vi "UI IDEX.vi"(8 "error in":errorcluster) -> (0 "error out":errorcluster)   [LabVIEW 2019, in "IDEX.lvlib"]
uses:
  IDEX.lvlib
  User Event/Controls/UE Abort Action.ctl
  <vilib>/Utility/miscctls.llb/LVPointTypeDef.ctl
  Queues/Queues.lvlib
panel:
  in  "Selection Valve":T1(ring)
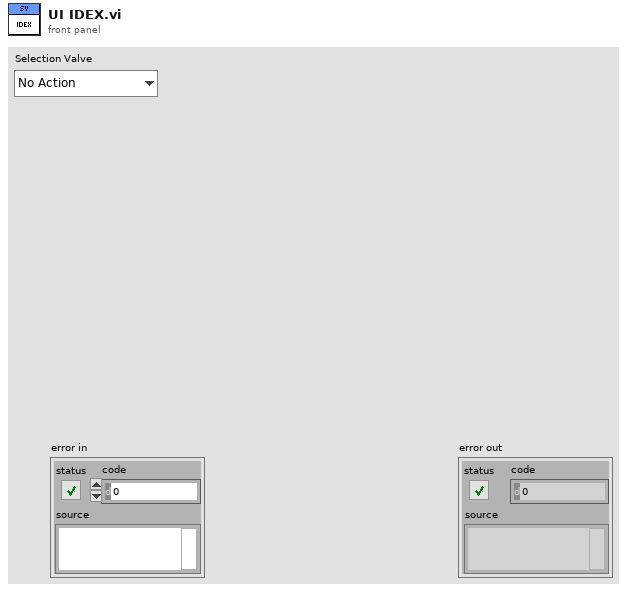
[diagram p1: front panel]
types:
  T1 = enum16{"No Action", "Position 1", "Position 2", "Position 3", "Position 4", "Position 5", "Position 6"}
  T2 = typedef "UE Abort Action.ctl" = enum16{"Create", "Get", "Destroy"}
  T3 = typedef "LVPointTypeDef.ctl" = cluster{"Horizontal":i16, "Vertical":i16}
  T4 = enum16{"Open", "Read", "Move", "Home", "Command", "Close"}
  T5 = typedef "IDEX.lvlib/SEQ Data.ctl" = cluster{"Position":string, "Initialize Done?":bool, "VI Refnum":refnum<vi>}
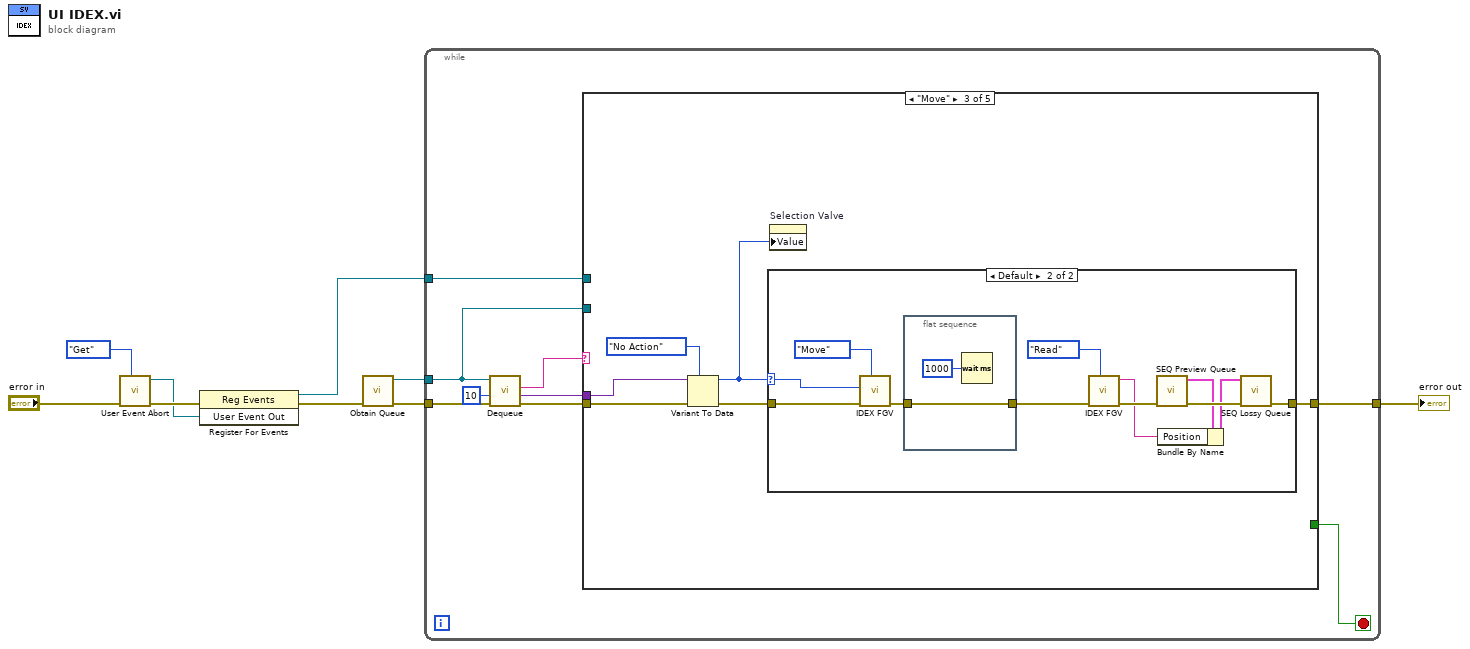
[diagram p0: block diagram]
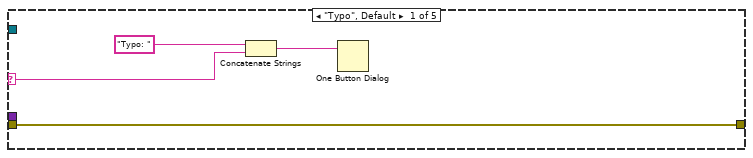
[diagram p2: hidden frame]
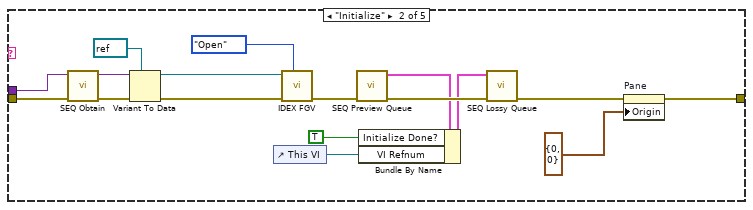
[diagram p3: hidden frame]
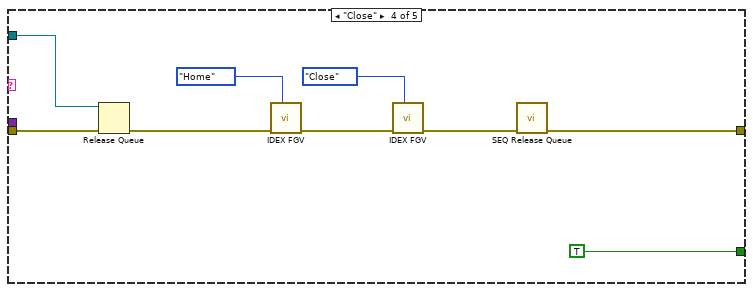
[diagram p5: hidden frame]
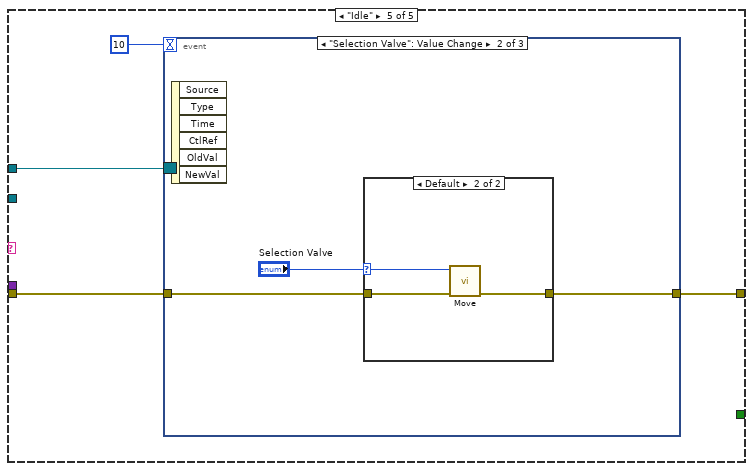
[diagram p6: hidden frame]
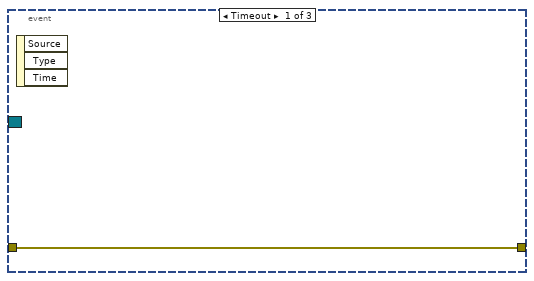
[diagram p7: hidden frame]
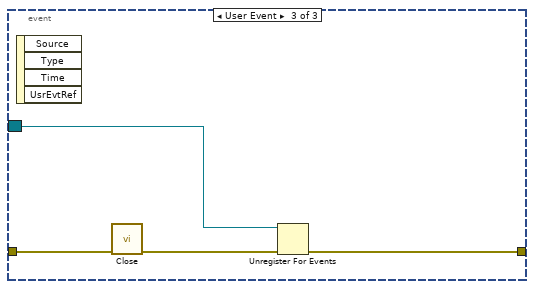
[diagram p9: hidden frame]
diagram:
  n1 = call "User Event Abort.vi"("Action"=UE_Abort_Action."Get", "Error In"="error in") -> ("Error Out"=w7:errorcluster, "User Event Out"=w6:refnum<user-event>)  [unwired: 8 in]
  n2 = register-events(error in=w7, w6) -> (reference out=w1:refnum<event-registration>, error out=w5:errorcluster)  [unwired: 1 in]
  n3 = call "Obtain Queue.vi"("Error In"=w5) -> ("Error Out"=w4:errorcluster, "Queue out"=w3:refnum<queue>)  [unwired: 9 in]
  n4 = while {
    tunnel: w4 -> [w18]
    tunnel: w3 -> [w13]
    tunnel: [w12] -> w2
    tunnel: w1 -> [w11]
    stop <- w10 stop-if-true
    n5 = call "Dequeue.vi"("Error In"=w18, "timeout in ms (-1)"=10, "Queue in"=w13) -> ("Error Out"=w17:errorcluster, "Data"=w15:variant, "State"=w16:string)  [unwired: 5 in, 1 out]
    n6 = case shown="\"Move\"" w16 {
      selector: w16 -> [w19 _ _ _ _]
      tunnel: w17 -> [w22 w32 w44 w68 w71]
      tunnel: w15 -> [_ w37 w43 _ _]
      tunnel: w13 -> [_ _ _ w67 _]
      tunnel: [w22 w25 w40 w60 w70] -> w12
      tunnel: w11 -> [_ _ _ _ w69]
      tunnel: [_ _ _ TRUE _] -> w10
      frame "Typo", Default {
        n7 = Concatenate Strings("Typo: " ("string"), w19) -> (w21:string)
        n8 = One Button Dialog(message=w21) -> ()  [unwired: 1 in, 1 out]
      }
      frame "Initialize" {
        n9 = call "SEQ Obtain.vi"("error in"=w32) -> ("error out"=w31:errorcluster)  [unwired: 9 in, 1 out]
        n10 = Variant To Data(error in=w31, type=refnum<visa-resource-name> refnum ("VISA resource name"), Variant=w37) -> (data=w35:refnum<visa-resource-name>, error out=w38:errorcluster)
        n11 = control-ref of="This VI"() -> (w23:refnum<vi>)
        n12 = call "IDEX FGV.vi"("Function"=T4."Open", "error in"=w38, "VISA resource name"=w35) -> ("error out"=w30:errorcluster)  [unwired: 7 in, 1 out]
        n13 = call "SEQ Preview Queue.vi"("error in"=w30) -> ("error out"=w33:errorcluster, "SEQ Data"=w29:T5)  [unwired: 9 in]
        n14 = Bundle By Name(cluster=w29, "Initialize Done?"=TRUE, "VI Refnum"=w23) -> (w28:T5)
        n15 = call "SEQ Lossy Queue.vi"("error in"=w33, "SEQ Data"=w28) -> ("error out"=w26:errorcluster)  [unwired: 9 in]
        n16 = property on="Pane" class="Pane"(error in=w26, "Origin"=T3 {"Horizontal"=0, "Vertical"=0}) -> (error out=w25:errorcluster)  [unwired: 1 in, 1 out]
      }
      frame "Move" {
        n17 = Variant To Data(error in=w44, type=T1."No Action" ("Position"), Variant=w43) -> (data=w39:T1, error out=w42:errorcluster)
        n18 = case shown="Default" w39 {
          selector: w39 -> [_ w46]
          tunnel: w42 -> [w45 w57]
          tunnel: [w45 w55] -> w40
          frame "No Action" {
          }
          frame Default {
            n19 = call "IDEX FGV.vi"("Function"=T4."Move", "error in"=w57, "Position"=w46) -> ("error out"=w48:errorcluster)  [unwired: 7 in, 1 out]
            n20 = flat-sequence {
              tunnel: w48 -> [w59]
              tunnel: [w59] -> w47
              frame #0 {
                n21 = Wait (ms)(milliseconds to wait=u32 1000) -> ()  [unwired: 1 out]
              }
            }
            n22 = call "IDEX FGV.vi"("Function"=T4."Read", "error in"=w47) -> ("error out"=w53:errorcluster, "Read String"=w49:string)  [unwired: 8 in]
            n23 = call "SEQ Preview Queue.vi"("error in"=w53) -> ("error out"=w52:errorcluster, "SEQ Data"=w51:T5)  [unwired: 9 in]
            n24 = Bundle By Name(cluster=w51, "Position"=w49) -> (w50:T5)
            n25 = call "SEQ Lossy Queue.vi"("error in"=w52, "SEQ Data"=w50) -> ("error out"=w55:errorcluster)  [unwired: 9 in]
          }
        }
        n26 = property on="Selection Valve" class="Enum (strict)"("Value"=w39) -> ()  [unwired: 2 in, 2 out]
      }
      frame "Close" {
        n27 = Release Queue(queue=w67, error in (no error)=w68) -> (error out=w65:errorcluster)  [unwired: 1 in, 2 out]
        n28 = call "IDEX FGV.vi"("Function"=T4."Home", "error in"=w65) -> ("error out"=w64:errorcluster)  [unwired: 8 in, 1 out]
        n29 = call "IDEX FGV.vi"("Function"=T4."Close", "error in"=w64) -> ("error out"=w61:errorcluster)  [unwired: 8 in, 1 out]
        n30 = call "SEQ Release Queue.vi"("error in"=w61) -> ("error out"=w60:errorcluster)  [unwired: 10 in]
      }
      frame "Idle" {
        n31 = event shown="[1] \"Selection Valve\": Value Change" {
          selector: w69 -> [_ _ w82]
          dyn-events: _ -> [_ _ _]
          timeout: 10 -> [_ _ _]
          tunnel: w71 -> [w73 w76 w84]
          tunnel: [w73 w75 w81] -> w70
          event Timeout {
            n32 = event-data() -> ()  [unwired: 1 in, 3 out]
          }
          event "Selection Valve": Value Change {
            n33 = event-data() -> ()  [unwired: 1 in, 6 out]
            n34 = case shown="Default" "Selection Valve" {
              selector: "Selection Valve" -> [_ w78]
              tunnel: w76 -> [w77 w80]
              tunnel: [w77 w79] -> w75
              frame "No Action" {
              }
              frame Default {
                n35 = call "Move.vi"("Error In"=w80, "Position"=w78) -> ("Error Out"=w79:errorcluster)  [unwired: 9 in]
              }
            }
          }
          event User Event {
            n36 = event-data() -> ()  [unwired: 1 in, 4 out]
            n37 = call "Close.vi"("Error In"=w84) -> ("Error Out"=w83:errorcluster)  [unwired: 10 in]
            n38 = Unregister For Events(event registration refnum=w82, error in=w83) -> (error out=w81:errorcluster)
          }
        }
      }
    }
  }
  "error out" <- w2
